vi "Filter Line with Prefix.vi"(0 "Functions in":T1[](array[typedef]), 1 "Prefix":string="//", 11 "error in (no error)":errorcluster) -> (4 "Functions":T1[](array[typedef]), 15 "error out":errorcluster)   [LabVIEW 2019]
uses:
  Line Details.ctl
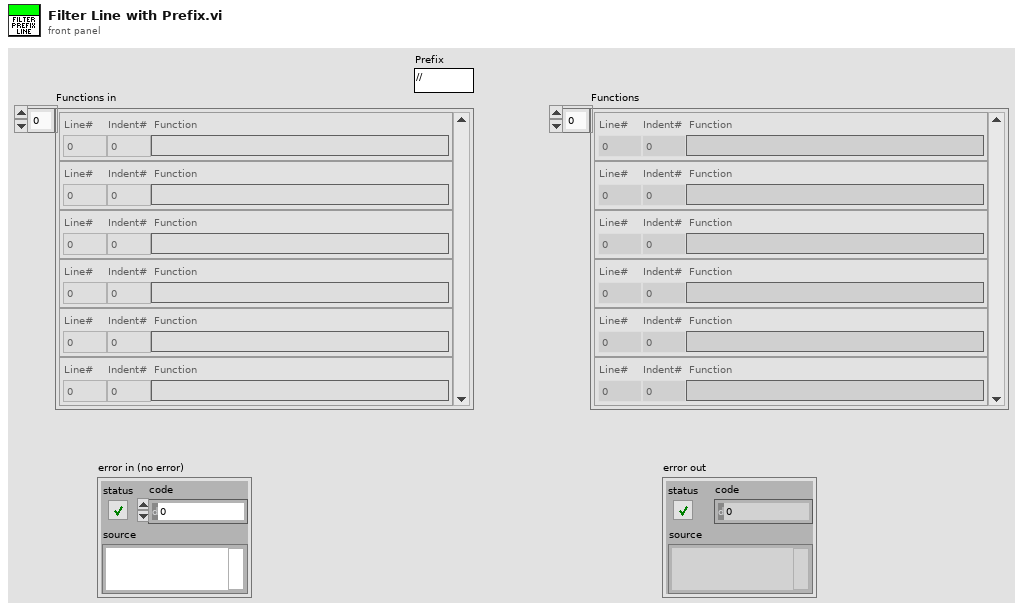
[diagram p1: front panel]
types:
  T1 = typedef "Line Details.ctl" = cluster{"Line#":i64, "Indent#":i64, "Function":string}
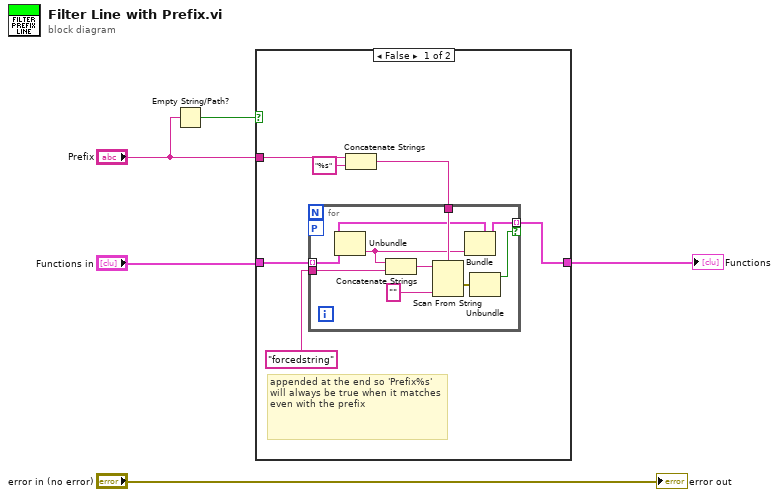
[diagram p0: block diagram]
diagram:
  n1 = Empty String/Path?(string/path="Prefix") -> (empty?=w4:bool)
  n2 = case shown="False" w4 {
    tunnel: "Functions in" -> [w9 w21]
    tunnel: [w8 w21] -> w2
    tunnel: "Prefix" -> [w7 _]
    frame False {
      # "appended at the end so 'Prefix%s' will always be true when it matches even with the prefix"
      n3 = Concatenate Strings(w7, "%s" ("string")) -> (w10:string)
      n4 = for {
        tunnel: w10 -> [w19]
        tunnel: w9 -> [w14] mode=indexing
        tunnel: [w13] -> w8 mode=indexing if=w17
        tunnel: "forcedstring" ("string") -> [w15]
        workers-P: _ -> [_]
        n5 = Unbundle(w14) -> ("Function"=w12:string)  [unwired: 2 out]
        n6 = Concatenate Strings(w12, w15) -> (w16:string)
        n7 = Scan From String(format string=w19, input string=w16, default 1="" ("string")) -> (error out=w18:errorcluster)  [unwired: 3 in, 2 out]
        n8 = Bundle(cluster=w14, "Function"=w12) -> (w13:T1)  [unwired: 2 in]
        n9 = Unbundle(w18) -> ("status"=w17:bool)  [unwired: 2 out]
      }
    }
    frame True {
    }
  }
  "Functions" <- w2
  "error out" <- "error in (no error)"
